vi "ToMotor1Command.vi"(9 "Encoder 1 count":i64, 10 "theta 0":i32, 11 "theta 1":i32) -> (2 "t":dbl, 3 "Boolean":bool)   [LabVIEW 2014]
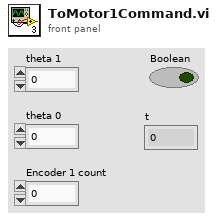
[diagram p1: front panel]
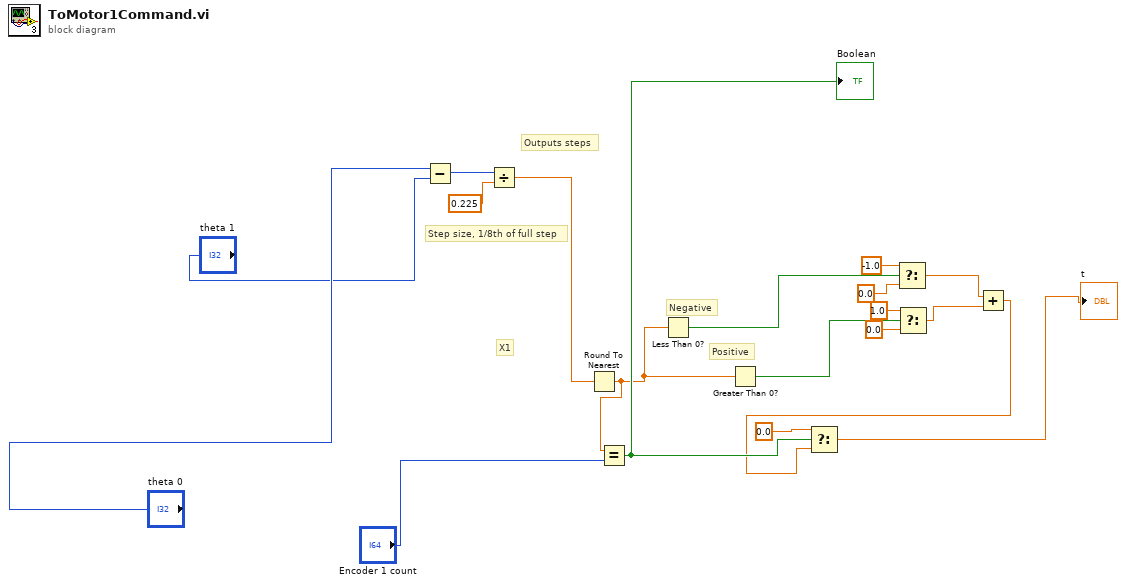
[diagram p0: block diagram]
diagram:
  # "Positive"
  # "Negative"
  # "Outputs steps"
  # "Step size, 1/8th of full step"
  # "X1"
  n1 = Subtract(x="theta 0", y="theta 1") -> (x-y=w2:i32)
  n2 = Divide(x=w2, y=0.225) -> (x/y=w4:dbl)
  n3 = Round To Nearest(number=w4) -> (nearest integer value=w14:dbl)
  n4 = Equal?(x=w14, y="Encoder 1 count") -> (x = y?=w19:bool)
  "Boolean" <- w19
  n5 = Less Than 0?(x=w14) -> (x < 0?=w7:bool)
  n6 = Greater Than 0?(x=w14) -> (x > 0?=w10:bool)
  n7 = Select(t=-1.0, s=w7, f=0.0) -> (s? t:f=w11:dbl)
  n8 = Select(t=1.0, s=w10, f=0.0) -> (s? t:f=w12:dbl)
  n9 = Add(x=w11, y=w12) -> (x+y=w16:dbl)
  n10 = Select(t=0.0, s=w19, f=w16) -> (s? t:f=→"t":dbl)
